vi "Send Data.vi"(8 "Detected Targets":T1(array[cluster]), 11 "name":string) -> ()   [LabVIEW 2015]
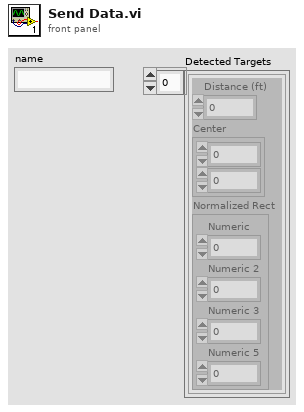
[diagram p1: front panel]
types:
  T1 = cluster{"Distance (ft)":dbl, "Center":cluster{dbl, dbl}, "Normalized Rect":cluster{"Numeric":dbl, "Numeric 2":dbl, "Numeric 3":dbl, "Numeric 5":dbl}}[]
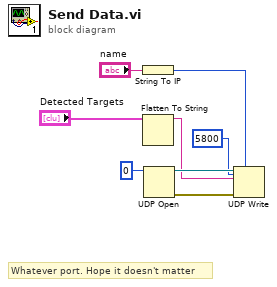
[diagram p0: block diagram]
diagram:
  # "Whatever port. Hope it doesn't matter"
  n1 = String To IP(1:"name") -> (0:w6:u32)
  n2 = Flatten To String(anything="Detected Targets") -> (data string=w3:string)  [unwired: 3 in, 2 out]
  n3 = UDP Open(11:u16 0 ("port")) -> (port=w8:refnum<k16>, 0:w7:errorcluster)  [unwired: 4 in, 1 out]
  n4 = UDP Write(address=w6, port or service name=u16 5800, connection ID=w8, data in=w3, 8:w7) -> ()  [unwired: 1 in, 2 out]
